vi "Set Variant.vi"(8 "error in (no error)":errorcluster, 10 "Variant (RFC)":T1=enum."RFC", 11 "UUID in":refnum<class "UUID.lvclass">) -> (0 "error out":errorcluster, 3 "UUID out":refnum<class "UUID.lvclass">)   [LabVIEW 2015, in "UUID.lvclass"]
uses:
  UUID.lvclass
  Variants.ctl
  UUID.lvclass/UUID.ctl
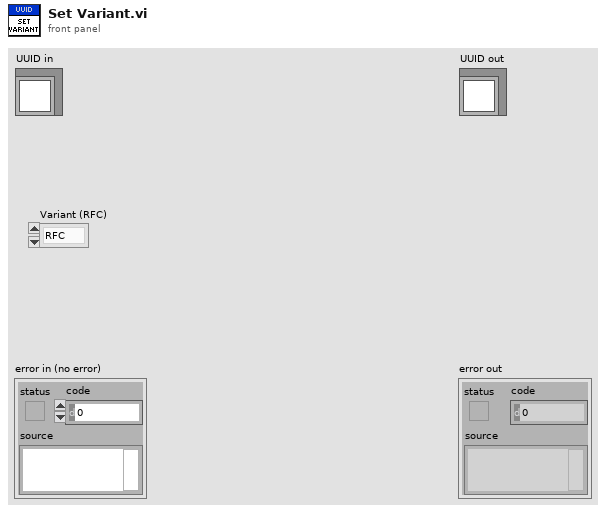
[diagram p1: front panel]
types:
  T1 = typedef "UUID.lvclass/Variants.ctl" = enum16{"NCS", "RFC", "Microsoft"}
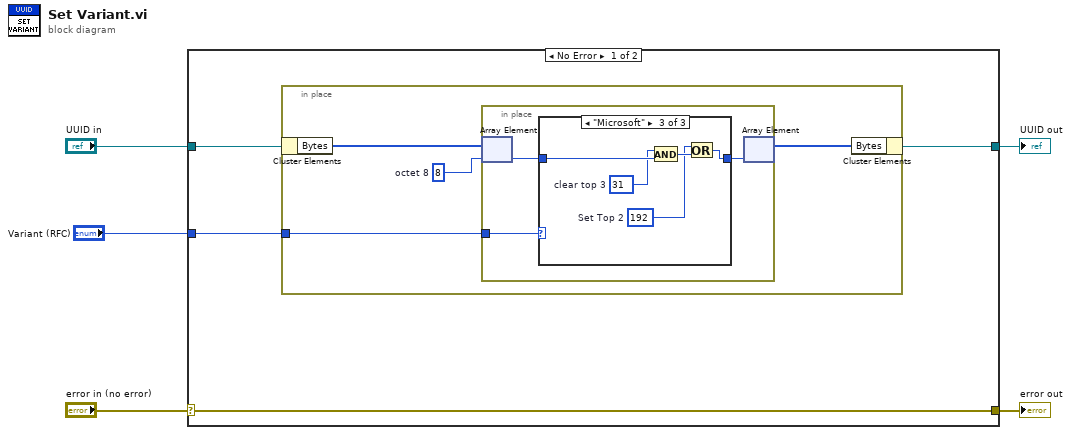
[diagram p0: block diagram]
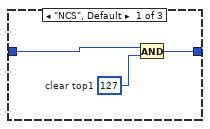
[diagram p2: hidden frame]
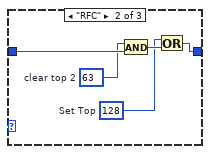
[diagram p3: hidden frame]
diagram:
  n1 = case shown="No Error" "error in (no error)" {
    selector: "error in (no error)" -> [w9 w31]
    tunnel: [w9 w31] -> w4
    tunnel: [w7 w30] -> w2
    tunnel: "UUID in" -> [w8 w30]
    tunnel: "Variant (RFC)" -> [w6 _]
    frame No Error {
      n2 = in-place {
        in-place-border: w6 -> [w10]
        w11 = 8  # octet 8
        n3 = in-place-cluster #1(w8) -> ("Bytes"=w13:u8[])
        n4 = in-place {
          in-place-border: w10 -> [w14]
          n5 = in-place-array #2(w13, w11) -> (w16:u8)
          n6 = case shown="\"Microsoft\"" w14 {
            tunnel: w16 -> [w19 w24 w29]
            tunnel: [w18 w23 w28] -> w15
            frame "NCS", Default {
              w17 = u8 127  # clear top1
              n7 = And(x=w19, y=w17) -> (x .and. y?=w18:u8)
            }
            frame "RFC" {
              w20 = u8 128  # Set Top
              w21 = u8 63  # clear top 2
              n8 = And(x=w21, y=w24) -> (x .and. y?=w22:u8)
              n9 = Or(x=w20, y=w22) -> (x .or. y?=w23:u8)
            }
            frame "Microsoft" {
              w25 = u8 192  # Set Top 2
              w26 = u8 31  # clear top 3
              n10 = And(x=w26, y=w29) -> (x .and. y?=w27:u8)
              n11 = Or(x=w25, y=w27) -> (x .or. y?=w28:u8)
            }
          }
          n12 = in-place-array #2(w15) -> (w12:u8[])  [unwired: 1 out]
        }
        n13 = in-place-cluster #1("Bytes"=w12) -> (w7:refnum<class "UUID.lvclass">)
      }
    }
    frame Error {
    }
  }
  "error out" <- w4
  "UUID out" <- w2
